vi "SP_OEE_2_test.vi"() -> ()   [LabVIEW 2017] (continued)
                        n399 = Format Into String(format string="Where BREAKDOWN_DATE between '%s' and '%s' and  SHIFT_ID = '%d'  ", w2102, w2100, w2088) -> (resulting string=w2099:string)  [unwired: 2 in, 1 out]
                        n400 = call <vilib>:"DB Tools Select Data.vi"("condition"=w2099, "error in (no error)"=w2108, "columns"=string[] ["BREAKDOWN_DATE"], "table"="STATION_1_LOG_HISTORY", "connection reference"=w2110) -> ("error out"=w2095:errorcluster, "data"=w2098:variant[][], "connection reference out"=w2109:T2)  [unwired: 1 in]
                        n401 = property on="Table 2" class="Tbl (strict)"("Visible"=FALSE) -> ()  [unwired: 2 in, 2 out]
                        n402 = xnode "Database Variant To Data"("database variant"=w2098, "error in (no error)"=w2095, "type"=string[][] [] ("Elements Found")) -> ("data"=w2096:string[][], "error out"=w2094:errorcluster)
                        n403 = Index Array(array=w2096, index (col)=0 ("disabled index (col)")) -> (element=w2104:string[])  [unwired: 1 in]
                        n404 = call "Search_1d_array_element.vi"("Count in"=string[] [] ("Elements Found"), "BD Date"=w2104, "Elements Found in"=string[] [] ("Elements Found")) -> ("Elements Found out"=w2091:string[])  [unwired: 4 in, 2 out]
                        n405 = Build Array(w2091) -> (w2114:string[][])
                        n406 = Transpose 2D Array(2D array=w2114) -> (transposed array=w2113:string[][])
                      }
                      frame #1 {
                        n407 = call "Stack_holderwise_total_bd_count_&_duration_2.vi"("Refnum in"=w2176, "BREAKDOWN_STK_HOLD_ID"=1, "condition"=w2163, "Form Date"=w2170, "To Date"=w2169, "error in (no error)"=w2174, "Shift"=w2160) -> ("Refnum out"=w2175:T2, "Count out"=w2168:string[], "appended array"=w2165:dbl[], "error out"=w2173:errorcluster)  [unwired: 5 in]
                        n408 = call "NUMERIC TO STRING.vi"("appended array"=w2165) -> ("Array"=w2164:string[])  [unwired: 4 in]
                        n409 = call "Insert_empty_element_with_zero.vi"("searched date"=w2168, "fixed date"=w2166) -> ("O/P"=w2161:string[])  [unwired: 9 in]
                        n410 = call "Insert_empty_element_with_zero.vi"("searched date"=w2164, "fixed date"=w2166) -> ("O/P"=w2167:string[])  [unwired: 9 in]
                      }
                      frame #2 {
                        n411 = disable-structure shown="Enabled" {
                          disable-tunnel: w2190 -> [w2203 w2205]
                          disable-tunnel: [w2202 w2205] -> w2189
                          disable-tunnel: w2188 -> [w2201 w2204]
                          disable-tunnel: [w2199 w2204] -> w2187
                          disable-tunnel: w2186 -> [w2198 _]
                          disable-tunnel: w2185 -> [w2197 _]
                          disable-tunnel: [w2196 _] -> w2184
                          disable-tunnel: [w2195 _] -> w2180
                          disable-tunnel: w2178 -> [w2194 _]
                          frame Disabled {
                            n412 = call "Stack_holderwise_total_bd_count_&_duration.vi"("Refnum in"=w2201, "BREAKDOWN_STK_HOLD_ID"=2, "condition"=w2194, "Form Date"=w2198, "To Date"=w2197, "error in (no error)"=w2203) -> ("Refnum out"=w2199:T2, "Count out"=w2196:string[], "appended array"=w2195:dbl[], "error out"=w2202:errorcluster)  [unwired: 6 in]
                          }
                          frame Enabled {
                          }
                        }
                        n413 = call "Insert_empty_element_with_zero.vi"("searched date"=w2184, "fixed date"=w2181) -> ("O/P"=w2183:string[])  [unwired: 9 in]
                        n414 = call "NUMERIC TO STRING.vi"("appended array"=w2180) -> ("Array"=w2179:string[])  [unwired: 4 in]
                        n415 = call "Insert_empty_element_with_zero.vi"("searched date"=w2179, "fixed date"=w2181) -> ("O/P"=w2182:string[])  [unwired: 9 in]
                      }
                      frame #3 {
                        n416 = disable-structure shown="Enabled" {
                          disable-tunnel: w2219 -> [w2233 w2236]
                          disable-tunnel: [w2232 w2236] -> w2218
                          disable-tunnel: w2217 -> [w2231 w2235]
                          disable-tunnel: [w2230 w2235] -> w2216
                          disable-tunnel: w2215 -> [w2229 _]
                          disable-tunnel: w2214 -> [w2228 _]
                          disable-tunnel: [w2227 _] -> w2213
                          disable-tunnel: [w2226 _] -> w2209
                          disable-tunnel: w2207 -> [w2225 _]
                          frame Disabled {
                            n417 = call "Stack_holderwise_total_bd_count_&_duration.vi"("Refnum in"=w2231, "BREAKDOWN_STK_HOLD_ID"=3, "condition"=w2225, "Form Date"=w2229, "To Date"=w2228, "error in (no error)"=w2233) -> ("Refnum out"=w2230:T2, "Count out"=w2227:string[], "appended array"=w2226:dbl[], "error out"=w2232:errorcluster)  [unwired: 6 in]
                          }
                          frame Enabled {
                          }
                        }
                        n418 = call "Insert_empty_element_with_zero.vi"("searched date"=w2213, "fixed date"=w2210) -> ("O/P"=w2212:string[])  [unwired: 9 in]
                        n419 = call "NUMERIC TO STRING.vi"("appended array"=w2209) -> ("Array"=w2208:string[])  [unwired: 4 in]
                        n420 = call "Insert_empty_element_with_zero.vi"("searched date"=w2208, "fixed date"=w2210) -> ("O/P"=w2211:string[])  [unwired: 9 in]
                      }
                      frame #4 {
                        n421 = disable-structure shown="Enabled" {
                          disable-tunnel: w2250 -> [w2266 w2269]
                          disable-tunnel: w2249 -> [w2265 w2268]
                          disable-tunnel: [w2264 w2268] -> w2248
                          disable-tunnel: [w2263 w2269] -> w2247
                          disable-tunnel: w2246 -> [w2262 _]
                          disable-tunnel: w2245 -> [w2261 _]
                          disable-tunnel: [w2260 _] -> w2244
                          disable-tunnel: [w2259 _] -> w2240
                          disable-tunnel: w2238 -> [w2258 _]
                          frame Disabled {
                            n422 = call "Stack_holderwise_total_bd_count_&_duration.vi"("Refnum in"=w2265, "BREAKDOWN_STK_HOLD_ID"=4, "condition"=w2258, "Form Date"=w2262, "To Date"=w2261, "error in (no error)"=w2266) -> ("Refnum out"=w2264:T2, "Count out"=w2260:string[], "appended array"=w2259:dbl[], "error out"=w2263:errorcluster)  [unwired: 6 in]
                          }
                          frame Enabled {
                          }
                        }
                        n423 = call "Insert_empty_element_with_zero.vi"("searched date"=w2244, "fixed date"=w2241) -> ("O/P"=w2243:string[])  [unwired: 9 in]
                        n424 = call "NUMERIC TO STRING.vi"("appended array"=w2240) -> ("Array"=w2239:string[])  [unwired: 4 in]
                        n425 = call "Insert_empty_element_with_zero.vi"("searched date"=w2239, "fixed date"=w2241) -> ("O/P"=w2242:string[])  [unwired: 9 in]
                      }
                      frame #5 {
                        n426 = disable-structure shown="Enabled" {
                          disable-tunnel: w2283 -> [w2301 w2304]
                          disable-tunnel: [w2300 w2304] -> w2282
                          disable-tunnel: w2281 -> [w2299 w2303]
                          disable-tunnel: [w2298 w2303] -> w2280
                          disable-tunnel: w2279 -> [w2297 _]
                          disable-tunnel: w2278 -> [w2296 _]
                          disable-tunnel: [w2295 _] -> w2277
                          disable-tunnel: [w2294 _] -> w2273
                          disable-tunnel: w2271 -> [w2293 _]
                          frame Disabled {
                            n427 = call "Stack_holderwise_total_bd_count_&_duration.vi"("Refnum in"=w2299, "BREAKDOWN_STK_HOLD_ID"=5, "condition"=w2293, "Form Date"=w2296, "To Date"=w2297, "error in (no error)"=w2301) -> ("Refnum out"=w2298:T2, "Count out"=w2295:string[], "appended array"=w2294:dbl[], "error out"=w2300:errorcluster)  [unwired: 6 in]
                          }
                          frame Enabled {
                          }
                        }
                        n428 = call "NUMERIC TO STRING.vi"("appended array"=w2273) -> ("Array"=w2272:string[])  [unwired: 4 in]
                        n429 = call "Insert_empty_element_with_zero.vi"("searched date"=w2277, "fixed date"=w2275) -> ("O/P"=w2276:string[])  [unwired: 9 in]
                        n430 = call "Insert_empty_element_with_zero.vi"("searched date"=w2272, "fixed date"=w2275) -> ("O/P"=w2274:string[])  [unwired: 9 in]
                      }
                      frame #6 {
                        n431 = call "String to numeric.vi"("Array"=w2315) -> ("Array 2"=w2314:dbl[])  [unwired: 4 in]
                        n432 = call "String to numeric.vi"("Array"=w2313) -> ("Array 2"=w2312:dbl[])  [unwired: 4 in]
                        n433 = call "String to numeric.vi"("Array"=w2311) -> ("Array 2"=w2310:dbl[])  [unwired: 4 in]
                        n434 = call "String to numeric.vi"("Array"=w2309) -> ("Array 2"=w2308:dbl[])  [unwired: 4 in]
                        n435 = call "String to numeric.vi"("Array"=w2307) -> ("Array 2"=w2306:dbl[])  [unwired: 4 in]
                        n436 = Decimal String To Number(string=w2320) -> (number=w2339:i32[])  [unwired: 2 in, 1 out]
                        n437 = Decimal String To Number(string=w2321) -> (number=w2340:i32[])  [unwired: 2 in, 1 out]
                        n438 = Decimal String To Number(string=w2322) -> (number=w2341:i32[])  [unwired: 2 in, 1 out]
                        n439 = Decimal String To Number(string=w2323) -> (number=w2342:i32[])  [unwired: 2 in, 1 out]
                        n440 = Decimal String To Number(string=w2324) -> (number=w2337:i32[])  [unwired: 2 in, 1 out]
                        n441 = Compound Arithmetic op=ADD(w2314, w2312, w2310, w2308, w2306) -> (w2317:dbl[])
                        n442 = Build Array(w2315) -> (w2336:string[][])
                        n443 = Build Array(w2313) -> (w2335:string[][])
                        n444 = Build Array(w2311) -> (w2334:string[][])
                        n445 = Build Array(w2309) -> (w2333:string[][])
                        n446 = Build Array(w2307) -> (w2332:string[][])
                        n447 = Number To Fractional String(number=w2317, precision (6)=i16 2) -> (F-format string=w2316:string[])  [unwired: 2 in]
                        n448 = Compound Arithmetic op=ADD(w2339, w2340, w2341, w2342, w2337) -> (w2343:i32[])
                        n449 = Transpose 2D Array(2D array=w2336) -> (transposed array=w2330:string[][])
                        n450 = Transpose 2D Array(2D array=w2335) -> (transposed array=w2329:string[][])
                        n451 = Transpose 2D Array(2D array=w2334) -> (transposed array=w2328:string[][])
                        n452 = Transpose 2D Array(2D array=w2333) -> (transposed array=w2327:string[][])
                        n453 = Transpose 2D Array(2D array=w2332) -> (transposed array=w2326:string[][])
                        n454 = Number To Decimal String(number=w2343) -> (decimal integer string=w2338:string[])  [unwired: 1 in]
                        n455 = Build Array(w2316) -> (w2319:string[][])
                        n456 = Transpose 2D Array(2D array=w2319) -> (transposed array=w2325:string[][])
                      }
                      frame #7 {
                        w2346 = string[] [""]
                        n457 = Insert Into Array(array=w2356, index (col)=1 ("disabled index (col)"), new element #1=w2355, new element #2=w2354, new element #3=w2346, new element #4=w2346, new element #5=w2346, new element #6=w2346, new element #7=w2346, new element #8=w2346, new element #9=w2346, new element #10=w2346, new element #11=w2347, new element #12=w2348) -> (w2350:string[][])  [unwired: 1 in]
                        n458 = call "flot graph for month n year.vi"("BD Date"=w2351, "error in (no error)"=w2353, "Count total"=w2347) -> ("error out"=w2352:errorcluster, "Run-Time Status"=w2349:cluster{"Array 2":timestamp[], dbl[]})  [unwired: 7 in]
                        n459 = local write "Run-Time Status"(w2349) -> ()
                        n460 = local write "Table"(w2350) -> ()
                      }
                    }
                  }
                  frame "2" {
                    n461 = flat-sequence {
                      tunnel: w2367 -> [w2481]
                      tunnel: w2366 -> [w2479]
                      tunnel: [w2465] -> w2457
                      tunnel: [w2480] -> w2456
                      tunnel: w2365 -> [_]
                      tunnel: [w2484] -> w2455
                      tunnel: [w2464] -> w2454
                      tunnel: [w2463] -> w2453
                      tunnel: [w2462] -> w2452
                      tunnel: w2364 -> [w2464]
                      tunnel: w2363 -> [w2463]
                      tunnel: ["Where BREAKDOWN_DATE between '%s'and '%s' and BREAKDOWN_STK_HOLD_ID ='%d' and  SHIFT_ID = '%d' "] -> w2451
                      tunnel: [w2462] -> w2450
                      tunnel: w2362 -> [w2458]
                      tunnel: [w2458] -> w2361
                      tunnel: w2457 -> [w2545]
                      tunnel: w2456 -> [w2547]
                      tunnel: w2455 -> [w2542]
                      tunnel: w2454 -> [w2541]
                      tunnel: w2453 -> [w2540]
                      tunnel: [w2544] -> w2449
                      tunnel: [w2546] -> w2448
                      tunnel: [w2542] -> w2447
                      tunnel: [w2532] -> w2446
                      tunnel: [w2538] -> w2445
                      tunnel: [w2541] -> w2444
                      tunnel: [w2540] -> w2443
                      tunnel: w2452 -> [w2537]
                      tunnel: [w2537] -> w2442
                      tunnel: w2451 -> [w2534]
                      tunnel: [w2534] -> w2441
                      tunnel: [w2533] -> w2440
                      tunnel: w2450 -> [w2533]
                      tunnel: w2361 -> [w2531]
                      tunnel: w2449 -> [w2561]
                      tunnel: w2448 -> [w2559]
                      tunnel: w2447 -> [w2564]
                      tunnel: w2446 -> [w2563]
                      tunnel: w2445 -> [w2562]
                      tunnel: w2444 -> [w2557]
                      tunnel: w2443 -> [w2556]
                      tunnel: [w2564] -> w2439
                      tunnel: [w2563] -> w2438
                      tunnel: [w2562] -> w2437
                      tunnel: [w2560] -> w2436
                      tunnel: [w2554] -> w2435
                      tunnel: [w2553] -> w2434
                      tunnel: [w2558] -> w2433
                      tunnel: [w2557] -> w2432
                      tunnel: [w2556] -> w2431
                      tunnel: w2442 -> [w2552]
                      tunnel: [w2552] -> w2430
                      tunnel: w2441 -> [w2549]
                      tunnel: [w2549] -> w2429
                      tunnel: [w2548] -> w2428
                      tunnel: w2440 -> [w2548]
                      tunnel: w2439 -> [w2595]
                      tunnel: w2438 -> [w2594]
                      tunnel: w2437 -> [w2593]
                      tunnel: w2436 -> [w2590]
                      tunnel: w2435 -> [w2592]
                      tunnel: w2434 -> [w2591]
                      tunnel: w2433 -> [w2588]
                      tunnel: w2432 -> [w2586]
                      tunnel: w2431 -> [w2585]
                      tunnel: [w2595] -> w2427
                      tunnel: [w2594] -> w2426
                      tunnel: [w2593] -> w2425
                      tunnel: [w2592] -> w2424
                      tunnel: [w2591] -> w2423
                      tunnel: [w2589] -> w2422
                      tunnel: [w2583] -> w2421
                      tunnel: [w2582] -> w2420
                      tunnel: [w2587] -> w2419
                      tunnel: [w2586] -> w2418
                      tunnel: [w2585] -> w2417
                      tunnel: w2430 -> [w2581]
                      tunnel: [w2581] -> w2416
                      tunnel: w2429 -> [w2578]
                      tunnel: [w2578] -> w2415
                      tunnel: [w2577] -> w2414
                      tunnel: w2428 -> [w2577]
                      tunnel: w2427 -> [w2628]
                      tunnel: w2426 -> [w2627]
                      tunnel: w2425 -> [w2626]
                      tunnel: w2424 -> [w2625]
                      tunnel: w2423 -> [w2624]
                      tunnel: w2422 -> [w2621]
                      tunnel: w2421 -> [w2623]
                      tunnel: w2420 -> [w2622]
                      tunnel: w2419 -> [w2620]
                      tunnel: w2418 -> [w2617]
                      tunnel: w2417 -> [w2616]
                      tunnel: [w2628] -> w2413
                      tunnel: [w2627] -> w2412
                      tunnel: [w2626] -> w2411
                      tunnel: [w2625] -> w2410
                      tunnel: [w2624] -> w2409
                      tunnel: [w2623] -> w2408
                      tunnel: [w2622] -> w2407
                      tunnel: [w2619] -> w2406
                      tunnel: [w2618] -> w2405
                      tunnel: [w2614] -> w2404
                      tunnel: [w2613] -> w2403
                      tunnel: [w2617] -> w2402
                      tunnel: [w2616] -> w2401
                      tunnel: w2416 -> [w2612]
                      tunnel: [w2612] -> w2400
                      tunnel: w2415 -> [w2609]
                      tunnel: [w2609] -> w2399
                      tunnel: [w2608] -> w2398
                      tunnel: w2414 -> [w2608]
                      tunnel: w2413 -> [w2663]
                      tunnel: w2412 -> [w2662]
                      tunnel: w2411 -> [w2661]
                      tunnel: w2410 -> [w2660]
                      tunnel: w2409 -> [w2659]
                      tunnel: w2408 -> [w2658]
                      tunnel: w2407 -> [w2657]
                      tunnel: w2406 -> [w2652]
                      tunnel: w2405 -> [w2654]
                      tunnel: w2404 -> [w2656]
                      tunnel: w2403 -> [w2655]
                      tunnel: w2402 -> [w2649]
                      tunnel: w2401 -> [w2650]
                      tunnel: [w2663] -> w2397
                      tunnel: [w2662] -> w2396
                      tunnel: [w2661] -> w2395
                      tunnel: [w2660] -> w2394
                      tunnel: [w2659] -> w2393
                      tunnel: [w2658] -> w2392
                      tunnel: [w2657] -> w2391
                      tunnel: [w2656] -> w2390
                      tunnel: [w2655] -> w2389
                      tunnel: [w2653] -> w2388
                      tunnel: [w2651] -> w2387
                      tunnel: [w2647] -> w2386
                      tunnel: [w2645] -> w2385
                      tunnel: w2400 -> [w2646]
                      tunnel: w2399 -> [w2642]
                      tunnel: [w2641] -> w2384
                      tunnel: w2398 -> [w2641]
                      tunnel: w2397 -> [w2702]
                      tunnel: w2396 -> [w2695]
                      tunnel: w2395 -> [w2686]
                      tunnel: w2394 -> [w2694]
                      tunnel: w2393 -> [w2684]
                      tunnel: w2392 -> [w2693]
                      tunnel: w2391 -> [w2682]
                      tunnel: w2390 -> [w2692]
                      tunnel: w2389 -> [w2680]
                      tunnel: w2388 -> [w2716]
                      tunnel: w2387 -> [w2715]
                      tunnel: w2386 -> [w2691]
                      tunnel: w2385 -> [w2678]
                      tunnel: [w2716] -> w2383
                      tunnel: [w2715] -> w2382
                      tunnel: [w2709] -> w2381
                      tunnel: [w2702] -> w2380
                      tunnel: [w2701] -> w2379
                      tunnel: [w2700] -> w2378
                      tunnel: [w2699] -> w2377
                      tunnel: [w2698] -> w2376
                      tunnel: [w2697] -> w2375
                      tunnel: [w2696] -> w2374
                      tunnel: [w2695] -> w2373
                      tunnel: [w2694] -> w2372
                      tunnel: [w2693] -> w2371
                      tunnel: [w2692] -> w2370
                      tunnel: [w2691] -> w2369
                      tunnel: [w2676] -> w2368
                      tunnel: w2384 -> [w2676]
                      tunnel: [w2729] -> w2359
                      tunnel: [w2723] -> w2360
                      tunnel: w2383 -> [w2724]
                      tunnel: w2382 -> [w2729]
                      tunnel: w2381 -> [w2718]
                      tunnel: w2380 -> [w2727]
                      tunnel: w2379 -> [w2725]
                      tunnel: w2378 -> [_]
                      tunnel: w2377 -> [_]
                      tunnel: w2376 -> [_]
                      tunnel: w2375 -> [_]
                      tunnel: w2374 -> [w2719]
                      tunnel: w2373 -> [w2726]
                      tunnel: w2372 -> [_]
                      tunnel: w2371 -> [_]
                      tunnel: w2370 -> [_]
                      tunnel: w2369 -> [_]
                      tunnel: w2368 -> [w2722]
                      frame #0 {
                        w2472 = "%Y-%m-%d" ("time format string (%c)")
                        n462 = Decimal String To Number(string=w2458) -> (number=w2459:i32)  [unwired: 2 in, 1 out]
                        n463 = property on="Table" class="Tbl (strict)"("Visible"=TRUE) -> ()  [unwired: 2 in, 2 out]
                        n464 = Format Date/Time String(time format string (%c)=w2472, seconds (now)=w2464) -> (date/time string=w2473:string)  [unwired: 1 in]
                        n465 = Format Date/Time String(time format string (%c)=w2472, seconds (now)=w2463) -> (date/time string=w2471:string)  [unwired: 1 in]
                        n466 = Format Into String(format string="Where BREAKDOWN_DATE between '%s' and '%s' and  SHIFT_ID = '%d'  ", w2473, w2471, w2459) -> (resulting string=w2470:string)  [unwired: 2 in, 1 out]
                        n467 = call <vilib>:"DB Tools Select Data.vi"("condition"=w2470, "error in (no error)"=w2479, "columns"=string[] ["BREAKDOWN_DATE"], "table"="STATION_1_LOG_HISTORY", "connection reference"=w2481) -> ("error out"=w2466:errorcluster, "data"=w2469:variant[][], "connection reference out"=w2480:T2)  [unwired: 1 in]
                        n468 = property on="Table 2" class="Tbl (strict)"("Visible"=FALSE) -> ()  [unwired: 2 in, 2 out]
                        n469 = xnode "Database Variant To Data"("database variant"=w2469, "error in (no error)"=w2466, "type"=string[][] [] ("Elements Found")) -> ("data"=w2467:string[][], "error out"=w2465:errorcluster)
                        n470 = Index Array(array=w2467, index (col)=0 ("disabled index (col)")) -> (element=w2475:string[])  [unwired: 1 in]
                        n471 = call "Search_1d_array_element.vi"("Count in"=string[] [] ("Elements Found"), "BD Date"=w2475, "Elements Found in"=string[] [] ("Elements Found")) -> ("Elements Found out"=w2462:string[])  [unwired: 4 in, 2 out]
                        n472 = Build Array(w2462) -> (w2485:string[][])
                        n473 = Transpose 2D Array(2D array=w2485) -> (transposed array=w2484:string[][])
                      }
                      frame #1 {
                        n474 = call "Stack_holderwise_total_bd_count_&_duration_2.vi"("Refnum in"=w2547, "BREAKDOWN_STK_HOLD_ID"=1, "condition"=w2534, "Form Date"=w2541, "To Date"=w2540, "error in (no error)"=w2545, "Shift"=w2531) -> ("Refnum out"=w2546:T2, "Count out"=w2539:string[], "appended array"=w2536:dbl[], "error out"=w2544:errorcluster)  [unwired: 5 in]
                        n475 = call "NUMERIC TO STRING.vi"("appended array"=w2536) -> ("Array"=w2535:string[])  [unwired: 4 in]
                        n476 = call "Insert_empty_element_with_zero.vi"("searched date"=w2539, "fixed date"=w2537) -> ("O/P"=w2532:string[])  [unwired: 9 in]
                        n477 = call "Insert_empty_element_with_zero.vi"("searched date"=w2535, "fixed date"=w2537) -> ("O/P"=w2538:string[])  [unwired: 9 in]
                      }
                      frame #2 {
                        n478 = disable-structure shown="Enabled" {
                          disable-tunnel: w2561 -> [w2574 w2576]
                          disable-tunnel: [w2573 w2576] -> w2560
                          disable-tunnel: w2559 -> [w2572 w2575]
                          disable-tunnel: [w2570 w2575] -> w2558
                          disable-tunnel: w2557 -> [w2569 _]
                          disable-tunnel: w2556 -> [w2568 _]
                          disable-tunnel: [w2567 _] -> w2555
                          disable-tunnel: [w2566 _] -> w2551
                          disable-tunnel: w2549 -> [w2565 _]
                          frame Disabled {
                            n479 = call "Stack_holderwise_total_bd_count_&_duration.vi"("Refnum in"=w2572, "BREAKDOWN_STK_HOLD_ID"=2, "condition"=w2565, "Form Date"=w2569, "To Date"=w2568, "error in (no error)"=w2574) -> ("Refnum out"=w2570:T2, "Count out"=w2567:string[], "appended array"=w2566:dbl[], "error out"=w2573:errorcluster)  [unwired: 6 in]
                          }
                          frame Enabled {
                          }
                        }
                        n480 = call "Insert_empty_element_with_zero.vi"("searched date"=w2555, "fixed date"=w2552) -> ("O/P"=w2554:string[])  [unwired: 9 in]
                        n481 = call "NUMERIC TO STRING.vi"("appended array"=w2551) -> ("Array"=w2550:string[])  [unwired: 4 in]
                        n482 = call "Insert_empty_element_with_zero.vi"("searched date"=w2550, "fixed date"=w2552) -> ("O/P"=w2553:string[])  [unwired: 9 in]
                      }
                      frame #3 {
                        n483 = disable-structure shown="Enabled" {
                          disable-tunnel: w2590 -> [w2604 w2607]
                          disable-tunnel: [w2603 w2607] -> w2589
                          disable-tunnel: w2588 -> [w2602 w2606]
                          disable-tunnel: [w2601 w2606] -> w2587
                          disable-tunnel: w2586 -> [w2600 _]
                          disable-tunnel: w2585 -> [w2599 _]
                          disable-tunnel: [w2598 _] -> w2584
                          disable-tunnel: [w2597 _] -> w2580
                          disable-tunnel: w2578 -> [w2596 _]
                          frame Disabled {
                            n484 = call "Stack_holderwise_total_bd_count_&_duration.vi"("Refnum in"=w2602, "BREAKDOWN_STK_HOLD_ID"=3, "condition"=w2596, "Form Date"=w2600, "To Date"=w2599, "error in (no error)"=w2604) -> ("Refnum out"=w2601:T2, "Count out"=w2598:string[], "appended array"=w2597:dbl[], "error out"=w2603:errorcluster)  [unwired: 6 in]
                          }
                          frame Enabled {
                          }
                        }
                        n485 = call "Insert_empty_element_with_zero.vi"("searched date"=w2584, "fixed date"=w2581) -> ("O/P"=w2583:string[])  [unwired: 9 in]
                        n486 = call "NUMERIC TO STRING.vi"("appended array"=w2580) -> ("Array"=w2579:string[])  [unwired: 4 in]
                        n487 = call "Insert_empty_element_with_zero.vi"("searched date"=w2579, "fixed date"=w2581) -> ("O/P"=w2582:string[])  [unwired: 9 in]
                      }
                      frame #4 {
                        n488 = disable-structure shown="Enabled" {
                          disable-tunnel: w2621 -> [w2637 w2640]
                          disable-tunnel: w2620 -> [w2636 w2639]
                          disable-tunnel: [w2635 w2639] -> w2619
                          disable-tunnel: [w2634 w2640] -> w2618
                          disable-tunnel: w2617 -> [w2633 _]
                          disable-tunnel: w2616 -> [w2632 _]
                          disable-tunnel: [w2631 _] -> w2615
                          disable-tunnel: [w2630 _] -> w2611
                          disable-tunnel: w2609 -> [w2629 _]
                          frame Disabled {
                            n489 = call "Stack_holderwise_total_bd_count_&_duration.vi"("Refnum in"=w2636, "BREAKDOWN_STK_HOLD_ID"=4, "condition"=w2629, "Form Date"=w2633, "To Date"=w2632, "error in (no error)"=w2637) -> ("Refnum out"=w2635:T2, "Count out"=w2631:string[], "appended array"=w2630:dbl[], "error out"=w2634:errorcluster)  [unwired: 6 in]
                          }
                          frame Enabled {
                          }
                        }
                        n490 = call "Insert_empty_element_with_zero.vi"("searched date"=w2615, "fixed date"=w2612) -> ("O/P"=w2614:string[])  [unwired: 9 in]
                        n491 = call "NUMERIC TO STRING.vi"("appended array"=w2611) -> ("Array"=w2610:string[])  [unwired: 4 in]
                        n492 = call "Insert_empty_element_with_zero.vi"("searched date"=w2610, "fixed date"=w2612) -> ("O/P"=w2613:string[])  [unwired: 9 in]
                      }
                      frame #5 {
                        n493 = disable-structure shown="Enabled" {
                          disable-tunnel: w2654 -> [w2672 w2675]
                          disable-tunnel: [w2671 w2675] -> w2653
                          disable-tunnel: w2652 -> [w2670 w2674]
                          disable-tunnel: [w2669 w2674] -> w2651
                          disable-tunnel: w2650 -> [w2668 _]
                          disable-tunnel: w2649 -> [w2667 _]
                          disable-tunnel: [w2666 _] -> w2648
                          disable-tunnel: [w2665 _] -> w2644
                          disable-tunnel: w2642 -> [w2664 _]
                          frame Disabled {
                            n494 = call "Stack_holderwise_total_bd_count_&_duration.vi"("Refnum in"=w2670, "BREAKDOWN_STK_HOLD_ID"=5, "condition"=w2664, "Form Date"=w2667, "To Date"=w2668, "error in (no error)"=w2672) -> ("Refnum out"=w2669:T2, "Count out"=w2666:string[], "appended array"=w2665:dbl[], "error out"=w2671:errorcluster)  [unwired: 6 in]
                          }
                          frame Enabled {
                          }
                        }
                        n495 = call "NUMERIC TO STRING.vi"("appended array"=w2644) -> ("Array"=w2643:string[])  [unwired: 4 in]
                        n496 = call "Insert_empty_element_with_zero.vi"("searched date"=w2648, "fixed date"=w2646) -> ("O/P"=w2647:string[])  [unwired: 9 in]
                        n497 = call "Insert_empty_element_with_zero.vi"("searched date"=w2643, "fixed date"=w2646) -> ("O/P"=w2645:string[])  [unwired: 9 in]
                      }
                      frame #6 {
                        n498 = call "String to numeric.vi"("Array"=w2686) -> ("Array 2"=w2685:dbl[])  [unwired: 4 in]
                        n499 = call "String to numeric.vi"("Array"=w2684) -> ("Array 2"=w2683:dbl[])  [unwired: 4 in]
                        n500 = call "String to numeric.vi"("Array"=w2682) -> ("Array 2"=w2681:dbl[])  [unwired: 4 in]
                        n501 = call "String to numeric.vi"("Array"=w2680) -> ("Array 2"=w2679:dbl[])  [unwired: 4 in]
                        n502 = call "String to numeric.vi"("Array"=w2678) -> ("Array 2"=w2677:dbl[])  [unwired: 4 in]
                        n503 = Decimal String To Number(string=w2691) -> (number=w2710:i32[])  [unwired: 2 in, 1 out]
                        n504 = Decimal String To Number(string=w2692) -> (number=w2711:i32[])  [unwired: 2 in, 1 out]
                        n505 = Decimal String To Number(string=w2693) -> (number=w2712:i32[])  [unwired: 2 in, 1 out]
                        n506 = Decimal String To Number(string=w2694) -> (number=w2713:i32[])  [unwired: 2 in, 1 out]
                        n507 = Decimal String To Number(string=w2695) -> (number=w2708:i32[])  [unwired: 2 in, 1 out]
                        n508 = Compound Arithmetic op=ADD(w2685, w2683, w2681, w2679, w2677) -> (w2688:dbl[])
                        n509 = Build Array(w2686) -> (w2707:string[][])
                        n510 = Build Array(w2684) -> (w2706:string[][])
                        n511 = Build Array(w2682) -> (w2705:string[][])
                        n512 = Build Array(w2680) -> (w2704:string[][])
                        n513 = Build Array(w2678) -> (w2703:string[][])
                        n514 = Number To Fractional String(number=w2688, precision (6)=i16 2) -> (F-format string=w2687:string[])  [unwired: 2 in]
                        n515 = Compound Arithmetic op=ADD(w2710, w2711, w2712, w2713, w2708) -> (w2714:i32[])
                        n516 = Transpose 2D Array(2D array=w2707) -> (transposed array=w2701:string[][])
                        n517 = Transpose 2D Array(2D array=w2706) -> (transposed array=w2700:string[][])
                        n518 = Transpose 2D Array(2D array=w2705) -> (transposed array=w2699:string[][])
                        n519 = Transpose 2D Array(2D array=w2704) -> (transposed array=w2698:string[][])
                        n520 = Transpose 2D Array(2D array=w2703) -> (transposed array=w2697:string[][])
                        n521 = Number To Decimal String(number=w2714) -> (decimal integer string=w2709:string[])  [unwired: 1 in]
                        n522 = Build Array(w2687) -> (w2690:string[][])
                        n523 = Transpose 2D Array(2D array=w2690) -> (transposed array=w2696:string[][])
                      }
                      frame #7 {
                        w2717 = string[] [""]
                        n524 = Insert Into Array(array=w2727, index (col)=1 ("disabled index (col)"), new element #1=w2726, new element #2=w2725, new element #3=w2717, new element #4=w2717, new element #5=w2717, new element #6=w2717, new element #7=w2717, new element #8=w2717, new element #9=w2717, new element #10=w2717, new element #11=w2718, new element #12=w2719) -> (w2721:string[][])  [unwired: 1 in]
                        n525 = call "flot graph for month n year.vi"("BD Date"=w2722, "error in (no error)"=w2724, "Count total"=w2718) -> ("error out"=w2723:errorcluster, "Run-Time Status"=w2720:cluster{"Array 2":timestamp[], dbl[]})  [unwired: 7 in]
                        n526 = local write "Run-Time Status"(w2720) -> ()
                        n527 = local write "Table"(w2721) -> ()
                      }
                    }
                  }
                  frame "3" {
                    n528 = flat-sequence {
                      tunnel: w2736 -> [w2850]
                      tunnel: w2735 -> [w2848]
                      tunnel: [w2834] -> w2826
                      tunnel: [w2849] -> w2825
                      tunnel: w2734 -> [_]
                      tunnel: [w2853] -> w2824
                      tunnel: [w2833] -> w2823
                      tunnel: [w2832] -> w2822
                      tunnel: [w2831] -> w2821
                      tunnel: w2733 -> [w2833]
                      tunnel: w2732 -> [w2832]
                      tunnel: ["Where BREAKDOWN_DATE between '%s'and '%s' and BREAKDOWN_STK_HOLD_ID ='%d' and  SHIFT_ID = '%d' "] -> w2820
                      tunnel: [w2831] -> w2819
                      tunnel: w2731 -> [w2827]
                      tunnel: [w2827] -> w2730
                      tunnel: w2826 -> [w2914]
                      tunnel: w2825 -> [w2916]
                      tunnel: w2824 -> [w2911]
                      tunnel: w2823 -> [w2910]
                      tunnel: w2822 -> [w2909]
                      tunnel: [w2913] -> w2818
                      tunnel: [w2915] -> w2817
                      tunnel: [w2911] -> w2816
                      tunnel: [w2901] -> w2815
                      tunnel: [w2907] -> w2814
                      tunnel: [w2910] -> w2813
                      tunnel: [w2909] -> w2812
                      tunnel: w2821 -> [w2906]
                      tunnel: [w2906] -> w2811
                      tunnel: w2820 -> [w2903]
                      tunnel: [w2903] -> w2810
                      tunnel: [w2902] -> w2809
                      tunnel: w2819 -> [w2902]
                      tunnel: w2730 -> [w2900]
                      tunnel: w2818 -> [w2930]
                      tunnel: w2817 -> [w2928]
                      tunnel: w2816 -> [w2933]
                      tunnel: w2815 -> [w2932]
                      tunnel: w2814 -> [w2931]
                      tunnel: w2813 -> [w2926]
                      tunnel: w2812 -> [w2925]
                      tunnel: [w2933] -> w2808
                      tunnel: [w2932] -> w2807
                      tunnel: [w2931] -> w2806
                      tunnel: [w2929] -> w2805
                      tunnel: [w2923] -> w2804
                      tunnel: [w2922] -> w2803
                      tunnel: [w2927] -> w2802
                      tunnel: [w2926] -> w2801
                      tunnel: [w2925] -> w2800
                      tunnel: w2811 -> [w2921]
                      tunnel: [w2921] -> w2799
                      tunnel: w2810 -> [w2918]
                      tunnel: [w2918] -> w2798
                      tunnel: [w2917] -> w2797
                      tunnel: w2809 -> [w2917]
                      tunnel: w2808 -> [w2964]
                      tunnel: w2807 -> [w2963]
                      tunnel: w2806 -> [w2962]
                      tunnel: w2805 -> [w2959]
                      tunnel: w2804 -> [w2961]
                      tunnel: w2803 -> [w2960]
                      tunnel: w2802 -> [w2957]
                      tunnel: w2801 -> [w2955]
                      tunnel: w2800 -> [w2954]
                      tunnel: [w2964] -> w2796
                      tunnel: [w2963] -> w2795
                      tunnel: [w2962] -> w2794
                      tunnel: [w2961] -> w2793
                      tunnel: [w2960] -> w2792
                      tunnel: [w2958] -> w2791
                      tunnel: [w2952] -> w2790
                      tunnel: [w2951] -> w2789
                      tunnel: [w2956] -> w2788
                      tunnel: [w2955] -> w2787
                      tunnel: [w2954] -> w2786
                      tunnel: w2799 -> [w2950]
                      tunnel: [w2950] -> w2785
                      tunnel: w2798 -> [w2947]
                      tunnel: [w2947] -> w2784
                      tunnel: [w2946] -> w2783
                      tunnel: w2797 -> [w2946]
                      tunnel: w2796 -> [w2997]
                      tunnel: w2795 -> [w2996]
                      tunnel: w2794 -> [w2995]
                      tunnel: w2793 -> [w2994]
                      tunnel: w2792 -> [w2993]
                      tunnel: w2791 -> [w2990]
                      tunnel: w2790 -> [w2992]
                      tunnel: w2789 -> [w2991]
                      tunnel: w2788 -> [w2989]
                      tunnel: w2787 -> [w2986]
                      tunnel: w2786 -> [w2985]
                      tunnel: [w2997] -> w2782
                      tunnel: [w2996] -> w2781
                      tunnel: [w2995] -> w2780
                      tunnel: [w2994] -> w2779
                      tunnel: [w2993] -> w2778
                      tunnel: [w2992] -> w2777
                      tunnel: [w2991] -> w2776
                      tunnel: [w2988] -> w2775
                      tunnel: [w2987] -> w2774
                      tunnel: [w2983] -> w2773
                      tunnel: [w2982] -> w2772
                      tunnel: [w2986] -> w2771
                      tunnel: [w2985] -> w2770
                      tunnel: w2785 -> [w2981]
                      tunnel: [w2981] -> w2769
                      tunnel: w2784 -> [w2978]
                      tunnel: [w2978] -> w2768
                      tunnel: [w2977] -> w2767
                      tunnel: w2783 -> [w2977]
                      tunnel: w2782 -> [w3032]
                      tunnel: w2781 -> [w3031]
                      tunnel: w2780 -> [w3030]
                      tunnel: w2779 -> [w3029]
                      tunnel: w2778 -> [w3028]
                      tunnel: w2777 -> [w3027]
                      tunnel: w2776 -> [w3026]
                      tunnel: w2775 -> [w3021]
                      tunnel: w2774 -> [w3023]
                      tunnel: w2773 -> [w3025]
                      tunnel: w2772 -> [w3024]
                      tunnel: w2771 -> [w3018]
                      tunnel: w2770 -> [w3019]
                      tunnel: [w3032] -> w2766
                      tunnel: [w3031] -> w2765
                      tunnel: [w3030] -> w2764
                      tunnel: [w3029] -> w2763
                      tunnel: [w3028] -> w2762
                      tunnel: [w3027] -> w2761
                      tunnel: [w3026] -> w2760
                      tunnel: [w3025] -> w2759
                      tunnel: [w3024] -> w2758
                      tunnel: [w3022] -> w2757
                      tunnel: [w3020] -> w2756
                      tunnel: [w3016] -> w2755
                      tunnel: [w3014] -> w2754
                      tunnel: w2769 -> [w3015]
                      tunnel: w2768 -> [w3011]
                      tunnel: [w3010] -> w2753
                      tunnel: w2767 -> [w3010]
                      tunnel: w2766 -> [w3071]
                      tunnel: w2765 -> [w3064]
                      tunnel: w2764 -> [w3055]
                      tunnel: w2763 -> [w3063]
                      tunnel: w2762 -> [w3053]
                      tunnel: w2761 -> [w3062]
                      tunnel: w2760 -> [w3051]
                      tunnel: w2759 -> [w3061]
                      tunnel: w2758 -> [w3049]
                      tunnel: w2757 -> [w3085]
                      tunnel: w2756 -> [w3084]
                      tunnel: w2755 -> [w3060]
                      tunnel: w2754 -> [w3047]
                      tunnel: [w3085] -> w2752
                      tunnel: [w3084] -> w2751
                      tunnel: [w3078] -> w2750
                      tunnel: [w3071] -> w2749
                      tunnel: [w3070] -> w2748
                      tunnel: [w3069] -> w2747
                      tunnel: [w3068] -> w2746
                      tunnel: [w3067] -> w2745
                      tunnel: [w3066] -> w2744
                      tunnel: [w3065] -> w2743
                      tunnel: [w3064] -> w2742
                      tunnel: [w3063] -> w2741
                      tunnel: [w3062] -> w2740
                      tunnel: [w3061] -> w2739
                      tunnel: [w3060] -> w2738
                      tunnel: [w3045] -> w2737
                      tunnel: w2753 -> [w3045]
                      tunnel: [w3098] -> _
                      tunnel: [w3092] -> _
                      tunnel: w2752 -> [w3093]
                      tunnel: w2751 -> [w3098]
                      tunnel: w2750 -> [w3087]
                      tunnel: w2749 -> [w3096]
                      tunnel: w2748 -> [w3094]
                      tunnel: w2747 -> [_]
                      tunnel: w2746 -> [_]
                      tunnel: w2745 -> [_]
                      tunnel: w2744 -> [_]
                      tunnel: w2743 -> [w3088]
                      tunnel: w2742 -> [w3095]
                      tunnel: w2741 -> [_]
                      tunnel: w2740 -> [_]
                      tunnel: w2739 -> [_]
                      tunnel: w2738 -> [_]
                      tunnel: w2737 -> [w3091]
                      frame #0 {
                        w2841 = "%Y-%m-%d" ("time format string (%c)")
                        n529 = Decimal String To Number(string=w2827) -> (number=w2828:i32)  [unwired: 2 in, 1 out]
                        n530 = property on="Table" class="Tbl (strict)"("Visible"=TRUE) -> ()  [unwired: 2 in, 2 out]
                        n531 = Format Date/Time String(time format string (%c)=w2841, seconds (now)=w2833) -> (date/time string=w2842:string)  [unwired: 1 in]
                        n532 = Format Date/Time String(time format string (%c)=w2841, seconds (now)=w2832) -> (date/time string=w2840:string)  [unwired: 1 in]
                        n533 = Format Into String(format string="Where BREAKDOWN_DATE between '%s' and '%s' and  SHIFT_ID = '%d'  ", w2842, w2840, w2828) -> (resulting string=w2839:string)  [unwired: 2 in, 1 out]
                        n534 = call <vilib>:"DB Tools Select Data.vi"("condition"=w2839, "error in (no error)"=w2848, "columns"=string[] ["BREAKDOWN_DATE"], "table"="STATION_1_LOG_HISTORY", "connection reference"=w2850) -> ("error out"=w2835:errorcluster, "data"=w2838:variant[][], "connection reference out"=w2849:T2)  [unwired: 1 in]
                        n535 = property on="Table 2" class="Tbl (strict)"("Visible"=FALSE) -> ()  [unwired: 2 in, 2 out]
                        n536 = xnode "Database Variant To Data"("database variant"=w2838, "error in (no error)"=w2835, "type"=string[][] [] ("Elements Found")) -> ("data"=w2836:string[][], "error out"=w2834:errorcluster)
                        n537 = Index Array(array=w2836, index (col)=0 ("disabled index (col)")) -> (element=w2844:string[])  [unwired: 1 in]
                        n538 = call "Search_1d_array_element.vi"("Count in"=string[] [] ("Elements Found"), "BD Date"=w2844, "Elements Found in"=string[] [] ("Elements Found")) -> ("Elements Found out"=w2831:string[])  [unwired: 4 in, 2 out]
                        n539 = Build Array(w2831) -> (w2854:string[][])
                        n540 = Transpose 2D Array(2D array=w2854) -> (transposed array=w2853:string[][])
                      }
                      frame #1 {
                        n541 = call "Stack_holderwise_total_bd_count_&_duration_2.vi"("Refnum in"=w2916, "BREAKDOWN_STK_HOLD_ID"=1, "condition"=w2903, "Form Date"=w2910, "To Date"=w2909, "error in (no error)"=w2914, "Shift"=w2900) -> ("Refnum out"=w2915:T2, "Count out"=w2908:string[], "appended array"=w2905:dbl[], "error out"=w2913:errorcluster)  [unwired: 5 in]
                        n542 = call "NUMERIC TO STRING.vi"("appended array"=w2905) -> ("Array"=w2904:string[])  [unwired: 4 in]
                        n543 = call "Insert_empty_element_with_zero.vi"("searched date"=w2908, "fixed date"=w2906) -> ("O/P"=w2901:string[])  [unwired: 9 in]
                        n544 = call "Insert_empty_element_with_zero.vi"("searched date"=w2904, "fixed date"=w2906) -> ("O/P"=w2907:string[])  [unwired: 9 in]
                      }
                      frame #2 {
                        n545 = disable-structure shown="Enabled" {
                          disable-tunnel: w2930 -> [w2943 w2945]
                          disable-tunnel: [w2942 w2945] -> w2929
                          disable-tunnel: w2928 -> [w2941 w2944]
                          disable-tunnel: [w2939 w2944] -> w2927
                          disable-tunnel: w2926 -> [w2938 _]
                          disable-tunnel: w2925 -> [w2937 _]
                          disable-tunnel: [w2936 _] -> w2924
                          disable-tunnel: [w2935 _] -> w2920
                          disable-tunnel: w2918 -> [w2934 _]
                          frame Disabled {
                            n546 = call "Stack_holderwise_total_bd_count_&_duration.vi"("Refnum in"=w2941, "BREAKDOWN_STK_HOLD_ID"=2, "condition"=w2934, "Form Date"=w2938, "To Date"=w2937, "error in (no error)"=w2943) -> ("Refnum out"=w2939:T2, "Count out"=w2936:string[], "appended array"=w2935:dbl[], "error out"=w2942:errorcluster)  [unwired: 6 in]
                          }
                          frame Enabled {
                          }
                        }
                        n547 = call "Insert_empty_element_with_zero.vi"("searched date"=w2924, "fixed date"=w2921) -> ("O/P"=w2923:string[])  [unwired: 9 in]
                        n548 = call "NUMERIC TO STRING.vi"("appended array"=w2920) -> ("Array"=w2919:string[])  [unwired: 4 in]
                        n549 = call "Insert_empty_element_with_zero.vi"("searched date"=w2919, "fixed date"=w2921) -> ("O/P"=w2922:string[])  [unwired: 9 in]
                      }
                      frame #3 {
                        n550 = disable-structure shown="Enabled" {
                          disable-tunnel: w2959 -> [w2973 w2976]
                          disable-tunnel: [w2972 w2976] -> w2958
                          disable-tunnel: w2957 -> [w2971 w2975]
                          disable-tunnel: [w2970 w2975] -> w2956
                          disable-tunnel: w2955 -> [w2969 _]
                          disable-tunnel: w2954 -> [w2968 _]
                          disable-tunnel: [w2967 _] -> w2953
                          disable-tunnel: [w2966 _] -> w2949
                          disable-tunnel: w2947 -> [w2965 _]
                          frame Disabled {
                            n551 = call "Stack_holderwise_total_bd_count_&_duration.vi"("Refnum in"=w2971, "BREAKDOWN_STK_HOLD_ID"=3, "condition"=w2965, "Form Date"=w2969, "To Date"=w2968, "error in (no error)"=w2973) -> ("Refnum out"=w2970:T2, "Count out"=w2967:string[], "appended array"=w2966:dbl[], "error out"=w2972:errorcluster)  [unwired: 6 in]
                          }
                          frame Enabled {
                          }
                        }
                        n552 = call "Insert_empty_element_with_zero.vi"("searched date"=w2953, "fixed date"=w2950) -> ("O/P"=w2952:string[])  [unwired: 9 in]
                        n553 = call "NUMERIC TO STRING.vi"("appended array"=w2949) -> ("Array"=w2948:string[])  [unwired: 4 in]
                        n554 = call "Insert_empty_element_with_zero.vi"("searched date"=w2948, "fixed date"=w2950) -> ("O/P"=w2951:string[])  [unwired: 9 in]
                      }
                      frame #4 {
                        n555 = disable-structure shown="Enabled" {
                          disable-tunnel: w2990 -> [w3006 w3009]
                          disable-tunnel: w2989 -> [w3005 w3008]
                          disable-tunnel: [w3004 w3008] -> w2988
                          disable-tunnel: [w3003 w3009] -> w2987
                          disable-tunnel: w2986 -> [w3002 _]
                          disable-tunnel: w2985 -> [w3001 _]
                          disable-tunnel: [w3000 _] -> w2984
                          disable-tunnel: [w2999 _] -> w2980
                          disable-tunnel: w2978 -> [w2998 _]
                          frame Disabled {
                            n556 = call "Stack_holderwise_total_bd_count_&_duration.vi"("Refnum in"=w3005, "BREAKDOWN_STK_HOLD_ID"=4, "condition"=w2998, "Form Date"=w3002, "To Date"=w3001, "error in (no error)"=w3006) -> ("Refnum out"=w3004:T2, "Count out"=w3000:string[], "appended array"=w2999:dbl[], "error out"=w3003:errorcluster)  [unwired: 6 in]
                          }
                          frame Enabled {
                          }
                        }
                        n557 = call "Insert_empty_element_with_zero.vi"("searched date"=w2984, "fixed date"=w2981) -> ("O/P"=w2983:string[])  [unwired: 9 in]
                        n558 = call "NUMERIC TO STRING.vi"("appended array"=w2980) -> ("Array"=w2979:string[])  [unwired: 4 in]
                        n559 = call "Insert_empty_element_with_zero.vi"("searched date"=w2979, "fixed date"=w2981) -> ("O/P"=w2982:string[])  [unwired: 9 in]
                      }
                      frame #5 {
                        n560 = disable-structure shown="Enabled" {
                          disable-tunnel: w3023 -> [w3041 w3044]
                          disable-tunnel: [w3040 w3044] -> w3022
                          disable-tunnel: w3021 -> [w3039 w3043]
                          disable-tunnel: [w3038 w3043] -> w3020
                          disable-tunnel: w3019 -> [w3037 _]
                          disable-tunnel: w3018 -> [w3036 _]
                          disable-tunnel: [w3035 _] -> w3017
                          disable-tunnel: [w3034 _] -> w3013
                          disable-tunnel: w3011 -> [w3033 _]
                          frame Disabled {
                            n561 = call "Stack_holderwise_total_bd_count_&_duration.vi"("Refnum in"=w3039, "BREAKDOWN_STK_HOLD_ID"=5, "condition"=w3033, "Form Date"=w3036, "To Date"=w3037, "error in (no error)"=w3041) -> ("Refnum out"=w3038:T2, "Count out"=w3035:string[], "appended array"=w3034:dbl[], "error out"=w3040:errorcluster)  [unwired: 6 in]
                          }
                          frame Enabled {
                          }
                        }
                        n562 = call "NUMERIC TO STRING.vi"("appended array"=w3013) -> ("Array"=w3012:string[])  [unwired: 4 in]
                        n563 = call "Insert_empty_element_with_zero.vi"("searched date"=w3017, "fixed date"=w3015) -> ("O/P"=w3016:string[])  [unwired: 9 in]
                        n564 = call "Insert_empty_element_with_zero.vi"("searched date"=w3012, "fixed date"=w3015) -> ("O/P"=w3014:string[])  [unwired: 9 in]
                      }
                      frame #6 {
                        n565 = call "String to numeric.vi"("Array"=w3055) -> ("Array 2"=w3054:dbl[])  [unwired: 4 in]
                        n566 = call "String to numeric.vi"("Array"=w3053) -> ("Array 2"=w3052:dbl[])  [unwired: 4 in]
                        n567 = call "String to numeric.vi"("Array"=w3051) -> ("Array 2"=w3050:dbl[])  [unwired: 4 in]
                        n568 = call "String to numeric.vi"("Array"=w3049) -> ("Array 2"=w3048:dbl[])  [unwired: 4 in]
                        n569 = call "String to numeric.vi"("Array"=w3047) -> ("Array 2"=w3046:dbl[])  [unwired: 4 in]
                        n570 = Decimal String To Number(string=w3060) -> (number=w3079:i32[])  [unwired: 2 in, 1 out]
                        n571 = Decimal String To Number(string=w3061) -> (number=w3080:i32[])  [unwired: 2 in, 1 out]
                        n572 = Decimal String To Number(string=w3062) -> (number=w3081:i32[])  [unwired: 2 in, 1 out]
                        n573 = Decimal String To Number(string=w3063) -> (number=w3082:i32[])  [unwired: 2 in, 1 out]
                        n574 = Decimal String To Number(string=w3064) -> (number=w3077:i32[])  [unwired: 2 in, 1 out]
                        n575 = Compound Arithmetic op=ADD(w3054, w3052, w3050, w3048, w3046) -> (w3057:dbl[])
                        n576 = Build Array(w3055) -> (w3076:string[][])
                        n577 = Build Array(w3053) -> (w3075:string[][])
                        n578 = Build Array(w3051) -> (w3074:string[][])
                        n579 = Build Array(w3049) -> (w3073:string[][])
                        n580 = Build Array(w3047) -> (w3072:string[][])
                        n581 = Number To Fractional String(number=w3057, precision (6)=i16 2) -> (F-format string=w3056:string[])  [unwired: 2 in]
                        n582 = Compound Arithmetic op=ADD(w3079, w3080, w3081, w3082, w3077) -> (w3083:i32[])
                        n583 = Transpose 2D Array(2D array=w3076) -> (transposed array=w3070:string[][])
                        n584 = Transpose 2D Array(2D array=w3075) -> (transposed array=w3069:string[][])
                        n585 = Transpose 2D Array(2D array=w3074) -> (transposed array=w3068:string[][])
                        n586 = Transpose 2D Array(2D array=w3073) -> (transposed array=w3067:string[][])
                        n587 = Transpose 2D Array(2D array=w3072) -> (transposed array=w3066:string[][])
                        n588 = Number To Decimal String(number=w3083) -> (decimal integer string=w3078:string[])  [unwired: 1 in]
                        n589 = Build Array(w3056) -> (w3059:string[][])
                        n590 = Transpose 2D Array(2D array=w3059) -> (transposed array=w3065:string[][])
                      }
                      frame #7 {
                        w3086 = string[] [""]
                        n591 = Insert Into Array(array=w3096, index (col)=1 ("disabled index (col)"), new element #1=w3095, new element #2=w3094, new element #3=w3086, new element #4=w3086, new element #5=w3086, new element #6=w3086, new element #7=w3086, new element #8=w3086, new element #9=w3086, new element #10=w3086, new element #11=w3087, new element #12=w3088) -> (w3090:string[][])  [unwired: 1 in]
                        n592 = call "flot graph for month n year.vi"("BD Date"=w3091, "error in (no error)"=w3093, "Count total"=w3087) -> ("error out"=w3092:errorcluster, "Run-Time Status"=w3089:cluster{"Array 2":timestamp[], dbl[]})  [unwired: 7 in]
                        n593 = local write "Run-Time Status"(w3089) -> ()
                        n594 = local write "Table"(w3090) -> ()
                      }
                    }
                  }
                }
              }
              frame "Logistics" {
                n595 = local read "Shift"() -> (w3101:string)
                n596 = case shown="\"3\"" w3101 {
                  selector: w3101 -> [_ w3475 w3851 w4227 _]
                  tunnel: w3106 -> [w3111 w3480 w3856 w4232 _]
                  tunnel: w3105 -> [w3110 w3479 w3855 w4231 _]
                  tunnel: w3104 -> [w3109 w3478 w3854 w4230 _]
                  tunnel: w3103 -> [w3108 w3477 w3853 w4229 _]
                  tunnel: w3102 -> [w3107 w3476 w3852 w4228 _]
                  tunnel: [_ w3472 w3848 w4223 _] -> w3100
                  tunnel: [_ w3471 w3847 w4224 _] -> w3099
                  frame "ALL", Default {
                    n597 = flat-sequence {
                      tunnel: w3111 -> [w3223]
                      tunnel: w3110 -> [w3221]
                      tunnel: [w3207] -> w3201
                      tunnel: [w3222] -> w3200
                      tunnel: w3109 -> [_]
                      tunnel: [w3226] -> w3199
                      tunnel: [w3206] -> w3198
                      tunnel: [w3205] -> w3197
                      tunnel: [w3203] -> w3196
                      tunnel: w3108 -> [w3206]
                      tunnel: w3107 -> [w3205]
                      tunnel: ["Where BREAKDOWN_DATE between '%s'and '%s' and BREAKDOWN_STK_HOLD_ID ='%d'  "] -> w3195
                      tunnel: [w3203] -> w3194
                      tunnel: w3201 -> [w3285]
                      tunnel: w3200 -> [w3287]
                      tunnel: w3199 -> [w3283]
                      tunnel: w3198 -> [w3282]
                      tunnel: w3197 -> [w3281]
                      tunnel: [w3284] -> w3193
                      tunnel: [w3286] -> w3192
                      tunnel: [w3283] -> w3191
                      tunnel: [w3273] -> w3190
                      tunnel: [w3279] -> w3189
                      tunnel: [w3282] -> w3188
                      tunnel: [w3281] -> w3187
                      tunnel: w3196 -> [w3278]
                      tunnel: [w3278] -> w3186
                      tunnel: w3195 -> [w3275]
                      tunnel: [w3275] -> w3185
                      tunnel: [w3274] -> w3184
                      tunnel: w3194 -> [w3274]
                      tunnel: w3193 -> [w3314]
                      tunnel: w3192 -> [w3312]
                      tunnel: w3191 -> [w3317]
                      tunnel: w3190 -> [w3316]
                      tunnel: w3189 -> [w3315]
                      tunnel: w3188 -> [w3310]
                      tunnel: w3187 -> [w3309]
                      tunnel: [w3317] -> w3183
                      tunnel: [w3316] -> w3182
                      tunnel: [w3315] -> w3181
                      tunnel: [w3313] -> w3180
                      tunnel: [w3307] -> w3179
                      tunnel: [w3306] -> w3178
                      tunnel: [w3311] -> w3177
                      tunnel: [w3310] -> w3176
                      tunnel: [w3309] -> w3175
                      tunnel: w3186 -> [w3305]
                      tunnel: [w3305] -> w3174
                      tunnel: w3185 -> [w3302]
                      tunnel: [w3302] -> w3173
                      tunnel: [w3301] -> w3172
                      tunnel: w3184 -> [w3301]
                      tunnel: w3183 -> [w3336]
                      tunnel: w3182 -> [w3335]
                      tunnel: w3181 -> [w3334]
                      tunnel: w3180 -> [w3331]
                      tunnel: w3179 -> [w3333]
                      tunnel: w3178 -> [w3332]
                      tunnel: w3177 -> [w3329]
                      tunnel: w3176 -> [w3327]
                      tunnel: w3175 -> [w3326]
                      tunnel: [w3336] -> w3171
                      tunnel: [w3335] -> w3170
                      tunnel: [w3334] -> w3169
                      tunnel: [w3333] -> w3168
                      tunnel: [w3332] -> w3167
                      tunnel: [w3330] -> w3166
                      tunnel: [w3324] -> w3165
                      tunnel: [w3323] -> w3164
                      tunnel: [w3328] -> w3163
                      tunnel: [w3327] -> w3162
                      tunnel: [w3326] -> w3161
                      tunnel: w3174 -> [w3322]
                      tunnel: [w3322] -> w3160
                      tunnel: w3173 -> [w3319]
                      tunnel: [w3319] -> w3159
                      tunnel: [w3318] -> w3158
                      tunnel: w3172 -> [w3318]
                      tunnel: w3171 -> [w3369]
                      tunnel: w3170 -> [w3368]
                      tunnel: w3169 -> [w3367]
                      tunnel: w3168 -> [w3366]
                      tunnel: w3167 -> [w3365]
                      tunnel: w3166 -> [w3362]
                      tunnel: w3165 -> [w3364]
                      tunnel: w3164 -> [w3363]
                      tunnel: w3163 -> [w3361]
                      tunnel: w3162 -> [w3358]
                      tunnel: w3161 -> [w3357]
                      tunnel: [w3369] -> w3157
                      tunnel: [w3368] -> w3156
                      tunnel: [w3367] -> w3155
                      tunnel: [w3366] -> w3154
                      tunnel: [w3365] -> w3153
                      tunnel: [w3364] -> w3152
                      tunnel: [w3363] -> w3151
                      tunnel: [w3360] -> w3150
                      tunnel: [w3359] -> w3149
                      tunnel: [w3355] -> w3148
                      tunnel: [w3354] -> w3147
                      tunnel: [w3358] -> w3146
                      tunnel: [w3357] -> w3145
                      tunnel: w3160 -> [w3353]
                      tunnel: [w3353] -> w3144
                      tunnel: w3159 -> [w3350]
                      tunnel: [w3350] -> w3143
                      tunnel: [w3349] -> w3142
                      tunnel: w3158 -> [w3349]
                      tunnel: w3157 -> [w3404]
                      tunnel: w3156 -> [w3403]
                      tunnel: w3155 -> [w3402]
                      tunnel: w3154 -> [w3401]
                      tunnel: w3153 -> [w3400]
                      tunnel: w3152 -> [w3399]
                      tunnel: w3151 -> [w3398]
                      tunnel: w3150 -> [w3393]
                      tunnel: w3149 -> [w3395]
                      tunnel: w3148 -> [w3397]
                      tunnel: w3147 -> [w3396]
                      tunnel: w3146 -> [w3390]
                      tunnel: w3145 -> [w3391]
                      tunnel: [w3404] -> w3141
                      tunnel: [w3403] -> w3140
                      tunnel: [w3402] -> w3139
                      tunnel: [w3401] -> w3138
                      tunnel: [w3400] -> w3137
                      tunnel: [w3399] -> w3136
                      tunnel: [w3398] -> w3135
                      tunnel: [w3397] -> w3134
                      tunnel: [w3396] -> w3133
                      tunnel: [w3394] -> w3132
                      tunnel: [w3392] -> w3131
                      tunnel: [w3388] -> w3130
                      tunnel: [w3386] -> w3129
                      tunnel: w3144 -> [w3387]
                      tunnel: w3143 -> [w3383]
                      tunnel: [w3382] -> w3128
                      tunnel: w3142 -> [w3382]
                      tunnel: w3141 -> [w3443]
                      tunnel: w3140 -> [w3436]
                      tunnel: w3139 -> [w3427]
                      tunnel: w3138 -> [w3435]
                      tunnel: w3137 -> [w3425]
                      tunnel: w3136 -> [w3434]
                      tunnel: w3135 -> [w3423]
                      tunnel: w3134 -> [w3433]
                      tunnel: w3133 -> [w3421]
                      tunnel: w3132 -> [w3457]
                      tunnel: w3131 -> [w3456]
                      tunnel: w3130 -> [w3432]
                      tunnel: w3129 -> [w3419]
                      tunnel: [w3457] -> w3127
                      tunnel: [w3456] -> w3126
                      tunnel: [w3450] -> w3125
                      tunnel: [w3443] -> w3124
                      tunnel: [w3442] -> w3123
                      tunnel: [w3441] -> w3122
                      tunnel: [w3440] -> w3121
                      tunnel: [w3439] -> w3120
                      tunnel: [w3438] -> w3119
                      tunnel: [w3437] -> w3118
                      tunnel: [w3436] -> w3117
                      tunnel: [w3435] -> w3116
                      tunnel: [w3434] -> w3115
                      tunnel: [w3433] -> w3114
                      tunnel: [w3432] -> w3113
                      tunnel: [w3417] -> w3112
                      tunnel: w3128 -> [w3417]
                      tunnel: [w3470] -> _
                      tunnel: [w3466] -> _
                      tunnel: w3127 -> [w3467]
                      tunnel: w3126 -> [w3470]
                      tunnel: w3125 -> [w3461]
                      tunnel: w3124 -> [w3468]
                      tunnel: w3123 -> [_]
                      tunnel: w3122 -> [w3459]
                      tunnel: w3121 -> [_]
                      tunnel: w3120 -> [_]
                      tunnel: w3119 -> [_]
                      tunnel: w3118 -> [w3462]
                      tunnel: w3117 -> [_]
                      tunnel: w3116 -> [w3460]
                      tunnel: w3115 -> [_]
                      tunnel: w3114 -> [_]
                      tunnel: w3113 -> [_]
                      tunnel: w3112 -> [w3465]
                      frame #0 {
                        w3214 = "%Y-%m-%d" ("time format string (%c)")
                        n598 = property on="Table" class="Tbl (strict)"("Visible"=TRUE) -> ()  [unwired: 2 in, 2 out]
                        n599 = Format Date/Time String(time format string (%c)=w3214, seconds (now)=w3206) -> (date/time string=w3215:string)  [unwired: 1 in]
                        n600 = Format Date/Time String(time format string (%c)=w3214, seconds (now)=w3205) -> (date/time string=w3213:string)  [unwired: 1 in]
                        n601 = Format Into String(format string="Where BREAKDOWN_DATE between '%s' and '%s' ", w3215, w3213) -> (resulting string=w3212:string)  [unwired: 2 in, 1 out]
                        n602 = call <vilib>:"DB Tools Select Data.vi"("condition"=w3212, "error in (no error)"=w3221, "columns"=string[] ["BREAKDOWN_DATE"], "table"="STATION_1_LOG_HISTORY", "connection reference"=w3223) -> ("error out"=w3208:errorcluster, "data"=w3211:variant[][], "connection reference out"=w3222:T2)  [unwired: 1 in]
                        n603 = property on="Table 2" class="Tbl (strict)"("Visible"=FALSE) -> ()  [unwired: 2 in, 2 out]
                        n604 = xnode "Database Variant To Data"("database variant"=w3211, "error in (no error)"=w3208, "type"=string[][] [] ("Elements Found")) -> ("data"=w3209:string[][], "error out"=w3207:errorcluster)
                        n605 = Index Array(array=w3209, index (col)=0 ("disabled index (col)")) -> (element=w3217:string[])  [unwired: 1 in]
                        n606 = call "Search_1d_array_element.vi"("Count in"=string[] [] ("Elements Found"), "BD Date"=w3217, "Elements Found in"=string[] [] ("Elements Found")) -> ("Elements Found out"=w3203:string[])  [unwired: 4 in, 2 out]
                        n607 = Build Array(w3203) -> (w3227:string[][])
                        n608 = Transpose 2D Array(2D array=w3227) -> (transposed array=w3226:string[][])
                      }
                      frame #1 {
                        n609 = disable-structure shown="Enabled" {
                          disable-tunnel: w3287 -> [w3297 w3298]
                          disable-tunnel: [w3296 w3298] -> w3286
                          disable-tunnel: w3285 -> [w3295 w3299]
                          disable-tunnel: [w3294 w3299] -> w3284
                          disable-tunnel: w3282 -> [w3292 _]
                          disable-tunnel: w3281 -> [w3291 _]
                          disable-tunnel: [w3290 _] -> w3280
                          disable-tunnel: [w3289 _] -> w3277
                          disable-tunnel: w3275 -> [w3288 _]
                          frame Disabled {
                            n610 = call "Stack_holderwise_total_bd_count_&_duration.vi"("Refnum in"=w3297, "BREAKDOWN_STK_HOLD_ID"=1, "condition"=w3288, "Form Date"=w3292, "To Date"=w3291, "error in (no error)"=w3295) -> ("Refnum out"=w3296:T2, "Count out"=w3290:string[], "appended array"=w3289:dbl[], "error out"=w3294:errorcluster)  [unwired: 6 in]
                          }
                          frame Enabled {
                          }
                        }
                        n611 = call "NUMERIC TO STRING.vi"("appended array"=w3277) -> ("Array"=w3276:string[])  [unwired: 4 in]
                        n612 = call "Insert_empty_element_with_zero.vi"("searched date"=w3280, "fixed date"=w3278) -> ("O/P"=w3273:string[])  [unwired: 9 in]
                        n613 = call "Insert_empty_element_with_zero.vi"("searched date"=w3276, "fixed date"=w3278) -> ("O/P"=w3279:string[])  [unwired: 9 in]
                      }
